vi "DatatoGraphChroma.vi"(0 "WaveformChartReference":refnum<vi>, 1 "PlotYScale":u32[](array[numeric]), 5 "WaveformArrayIn":waveform(dbl)[](array[waveform]), 11 "error in (no error)":errorcluster) -> (4 "WaveformArrayOut":waveform(dbl)[](array[waveform]), 6 "OutputString":string, 8 "Incorrect DataType?":bool, 15 "error out":errorcluster)   [LabVIEW 2018]
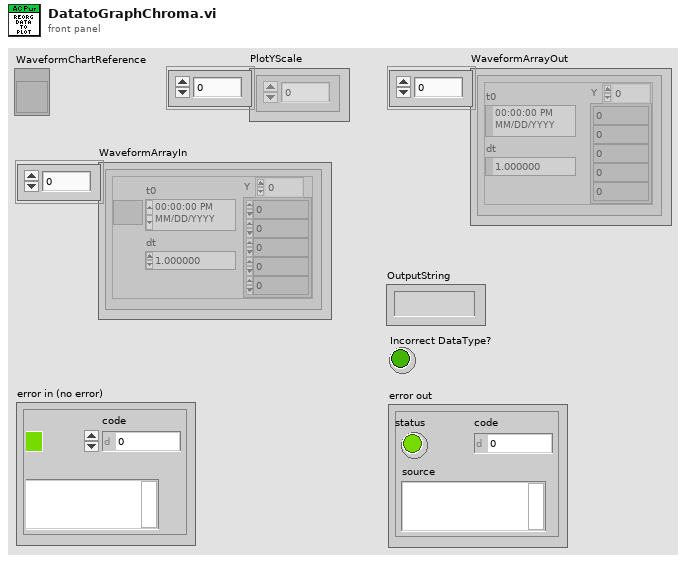
[diagram p1: front panel]
types:
  T1 = cluster{bool, "format string":string, "format string 2":string}
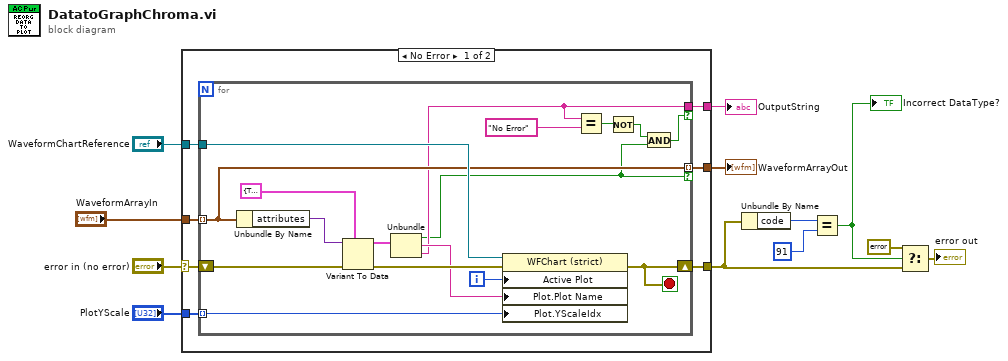
[diagram p0: block diagram]
diagram:
  n1 = case shown="No Error" "error in (no error)" {
    selector: "error in (no error)" -> [w19 w37]
    tunnel: [w18 w37] -> w3
    tunnel: [w17 _] -> w2
    tunnel: "WaveformChartReference" -> [w14 _]
    tunnel: "PlotYScale" -> [w16 _]
    tunnel: [w15 _] -> w9
    tunnel: "WaveformArrayIn" -> [w13 _]
    frame No Error {
      n2 = for {
        shift-right: [w33] -> w18
        shift-left: w19 -> [w26]
        tunnel: [w29] -> w17 mode=indexing if=w20
        tunnel: w14 -> [w35]
        tunnel: w16 -> [w34] mode=indexing
        tunnel: [w22] -> w15 if=w21
        tunnel: w13 -> [w29] mode=indexing
        i -> [w36]
        stop <- w33 stop-if-true
        n3 = Unbundle By Name(w29) -> ("attributes"=w28:variant)
        n4 = Variant To Data(error in=w26, type=T1 {TRUE, "format string"="%s", "format string 2"="%s"}, Variant=w28) -> (data=w24:T1, error out=w25:errorcluster)
        n5 = Unbundle(w24) -> (w20:bool, "format string"=w23:string, "format string 2"=w22:string)
        n6 = property on="Property Node" class="WFChart (strict)"(reference=w35, error in=w25, "Active Plot"=w36, "Plot.Plot Name"=w23, "Plot.YScaleIdx"=w34) -> (error out=w33:errorcluster)  [unwired: 1 out]
        n7 = Equal?(x=w22, y="No Error") -> (x = y?=w32:bool)
        n8 = Not(x=w32) -> (.not. x?=w31:bool)
        n9 = And(x=w31, y=w20) -> (x .and. y?=w21:bool)
      }
    }
    frame Error {
    }
  }
  "OutputString" <- w9
  "WaveformArrayOut" <- w2
  n10 = Unbundle By Name(w3) -> ("code"=w8:i32)
  n11 = Equal?(x=w8, y=91) -> (x = y?=w6:bool)
  "Incorrect DataType?" <- w6
  n12 = Select(t=errorcluster {"status"=FALSE, "code"=0, "source"=""} ("error IO"), s=w6, f=w3) -> (s? t:f=→"error out":errorcluster)
